vi "Determine Warnings.vi"() -> ()   [LabVIEW 2014]
panel:
  out "warning?":bool
  out "warning text":string
  in  "min temp":dbl
  in  "max temp":dbl
  in  "current temp":dbl
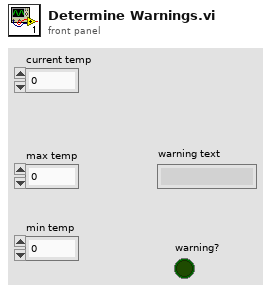
[diagram p1: front panel]
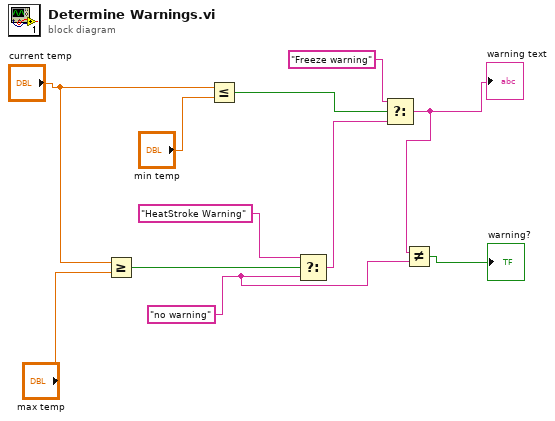
[diagram p0: block diagram]
diagram:
  w5 = "no warning"
  n1 = Greater Or Equal?(x="current temp", y="max temp") -> (x >= y?=w7:bool)
  n2 = Less Or Equal?(x="current temp", y="min temp") -> (x <= y?=w4:bool)
  n3 = Select(t="HeatStroke Warning", s=w7, f=w5) -> (s? t:f=w2:string)
  n4 = Select(t="Freeze warning", s=w4, f=w2) -> (s? t:f=w1:string)
  "warning text" <- w1
  n5 = Not Equal?(x=w1, y=w5) -> (x != y?=→"warning?":bool)
